vi "TRITON_SEND_RECEIVE.vi"(2 "error in (no error)":errorcluster, 3 "Command String":string, 4 "connection ID":refnum<k5>, 5 "Communication Cluster":T1) -> (0 "error out":errorcluster, 1 "Response String":string)   [LabVIEW 2015]
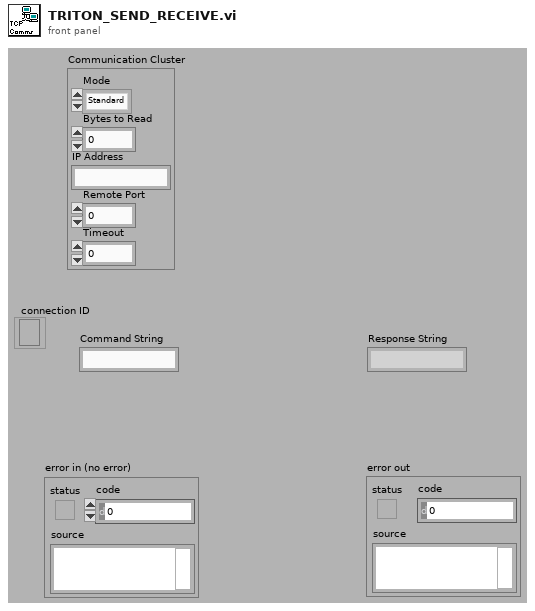
[diagram p1: front panel]
types:
  T1 = cluster{"Mode":enum16{"Standard", "Buffered", "CRLF", "Immediate"}, "Bytes to Read":i32, "IP Address":string, "Remote Port":i32, "Timeout":i32}
  T2 = enum16{"Standard", "Buffered", "CRLF", "Immediate"}
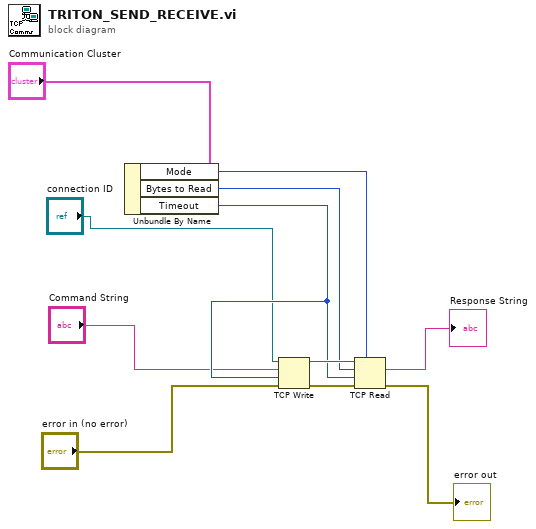
[diagram p0: block diagram]
diagram:
  n1 = Unbundle By Name("Communication Cluster") -> ("Mode"=w7:T2, "Bytes to Read"=w8:i32, "Timeout"=w9:i32)
  n2 = TCP Write(connection ID="connection ID", data in="Command String", error in (no error)="error in (no error)", 9:w9) -> (connection ID out=w10:refnum<k5>, error out=w11:errorcluster)  [unwired: 1 out]
  n3 = TCP Read(connection ID=w10, bytes to read=w8, error in (no error)=w11, 7:w7, 9:w9) -> (data out=→"Response String":string, error out=→"error out":errorcluster)  [unwired: 1 out]
